vi "Main.vi"() -> ()   [LabVIEW 2019]
uses:
  Main_state_enum.ctl
  Uart_codes_enum.ctl
  <vilib>/Instr/_visa.llb/VISA Configure Serial Port (Instr).vi
  <vilib>/Utility/file.llb/Write Delimited Spreadsheet (string).vi
panel:
  out "Polling error tips":string
  out "Serial error tips":string
  out "Blocker":string
  out "File path":path
  in  "Seconds":i32 caption="s" min=0 max=59 step=1
  in  "Minutes":i32 caption="m" min=0 max=59 step=1
  in  "Hours":i32 caption="h" min=0 max=23 step=1
  out "Cycle string":string caption="Automatic polling interval"
  out "Next reading in":string
  in  "Demo":bool caption="Frige/Freezer critical failure demo"
  in  "Manual read":bool caption="Reset serial or filename"
  out "Slide":dbl(slide) scale=0.0..3.0
  out "Demo indicator":bool
  out "Freezer alarm":bool
  out "Fridge alarm":bool
  out "AVG":dbl format="%#_4g"
  in  "Continue":bool caption="Reset serial or filename"
  in  "Filename":string
  out "Trend graph":cluster{i32, dbl}[](graph) caption="Average indoors temperature (Last 30 readings)"
  out "Trend":dbl[](array[numeric])
  out "Fridge warning":string
  out "Freezer warning":string
  out "FreezerSTR":string caption="Freezer"
  out "FridgeSTR":string caption="Fridge"
  out "BathroomSTR":string caption="Bathroom"
  out "LivingroomSTR":string caption="Livingroom"
  out "BedroomSTR":string caption="Bedroom"
  out "KitchenSTR":string caption="Kitchen"
  out "Last reading":string
  out "Current time":string
  out "Freezer":dbl(slide) scale=-18.0..-10.0 scale format="%#_2g"
  out "Fridge":dbl(slide) scale=3.0..6.0
  out "Bathroom":dbl(slide) scale=16.0..30.0
  out "Livingroom":dbl(slide) scale=16.0..30.0
  out "Bedroom":dbl(slide) scale=16.0..30.0
  out "Kitchen":dbl(slide) scale=16.0..30.0
  out "Outdoors":dbl(slide) scale=-30.0..30.0
  out "Reading Cycle(s)":i32=15
  out "UI show array":dbl[](array[numeric])=[6.0, 13.0, 24.0, 20.0, 21.0, 24.0, 4.0, -17.0]
  in  "insert_comport":refnum<visa-resource-name>="COM5" caption="Serial port"
  out "csv save array":string[](array[string])
  in  "stop":bool
  out "OutdoorsSTR":string caption="Outdoors"
  out "Floorplan":picture
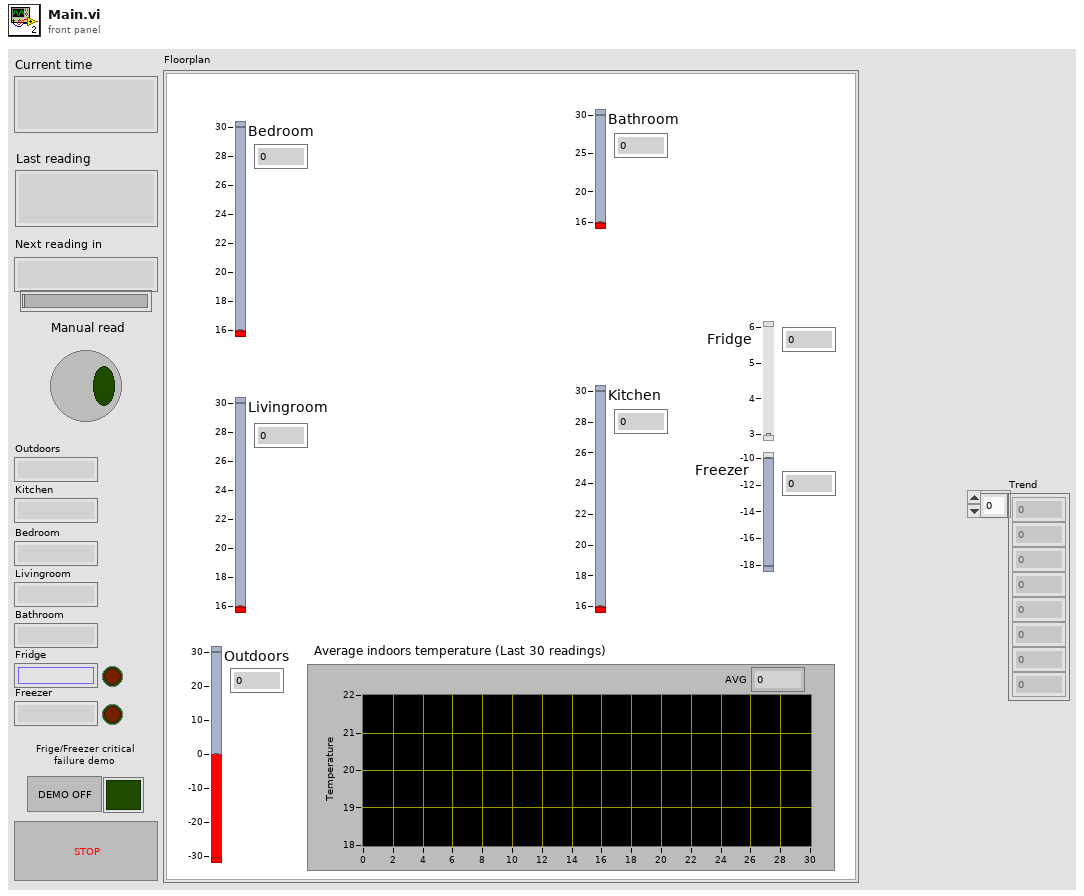
[diagram p1: front panel]
types:
  T1 = typedef "Uart_codes_enum.ctl" = enum16{"GET_READINGS", "FRIDGE_FREEZER_FAIL"}
  T2 = typedef "Main_state_enum.ctl" = enum16{"Init", "Set_startup_config", "Check_startup_config", "Read_serial", "Check_serial", "Update", "Wait"}
  T3 = enum8{"Enabled", "Disabled", "Disabled and Grayed Out"}
  T4 = typedef "imagedata.ctl" = cluster{"image type":i32, "image depth":i32, "image":u8[], "mask":u8[], "colors":u32[], "Rectangle":cluster{"left":i16, "top":i16, "right":i16, "bottom":i16}}
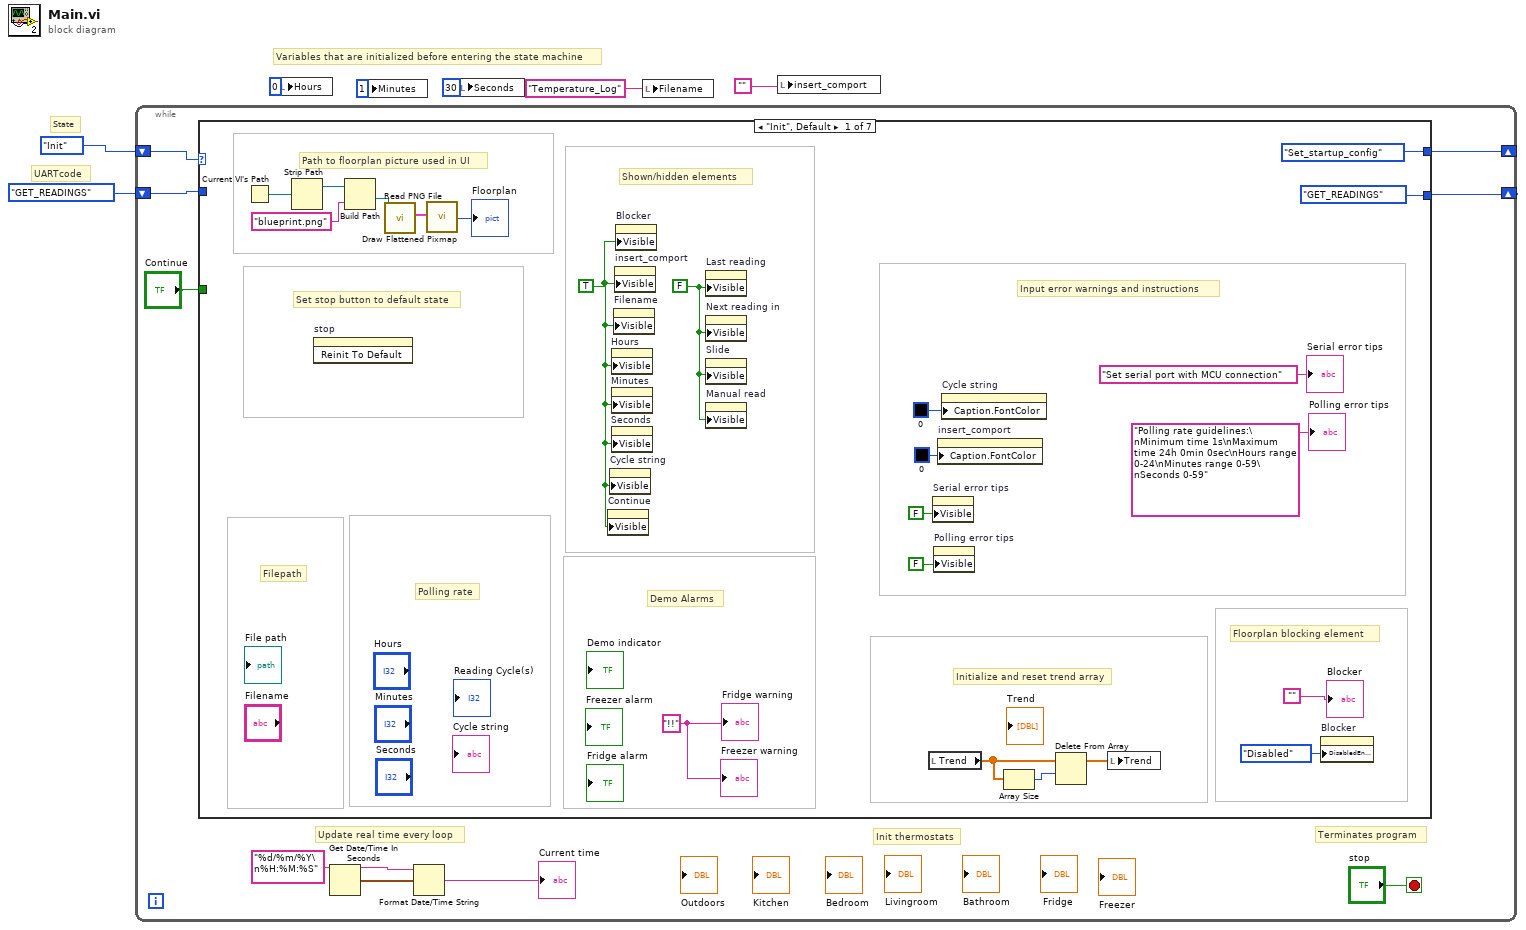
[diagram p0: block diagram]
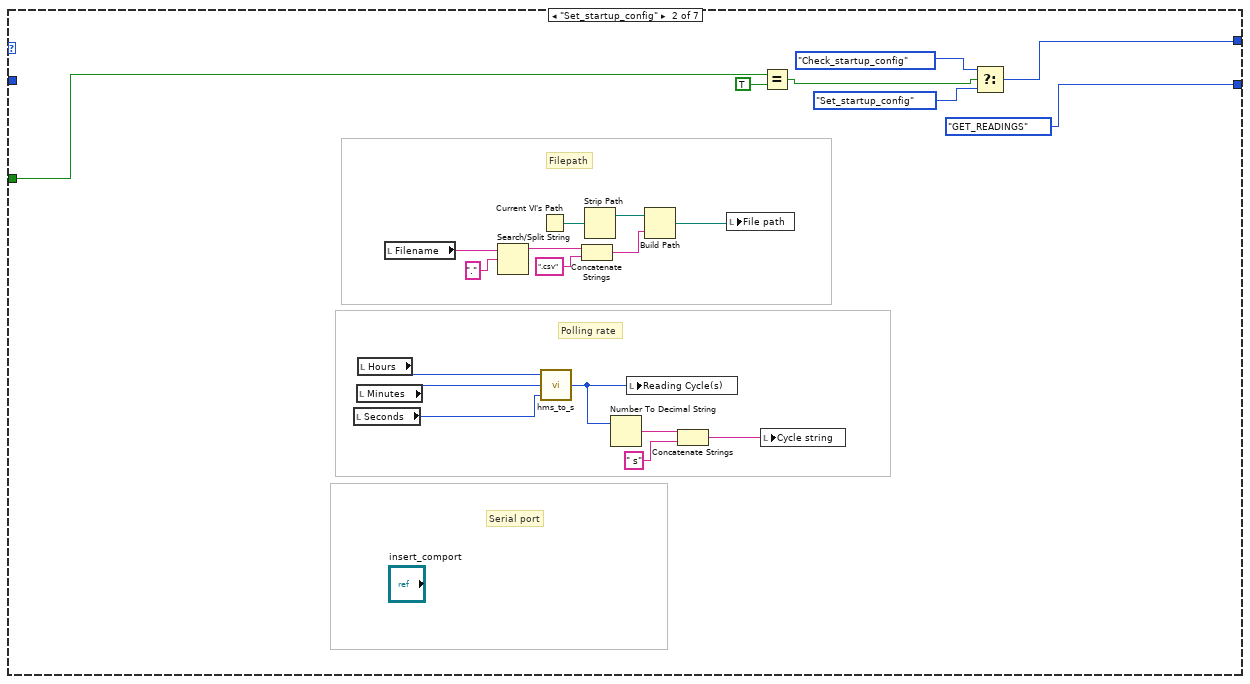
[diagram p2: hidden frame]
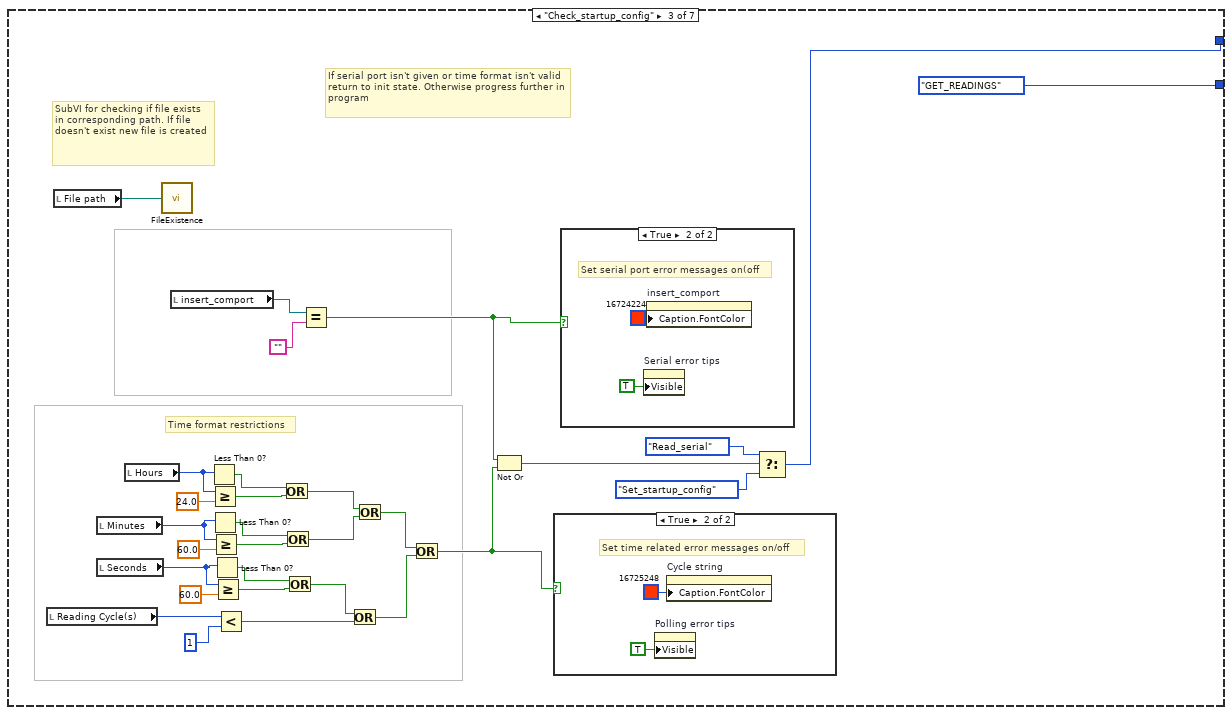
[diagram p3: hidden frame]
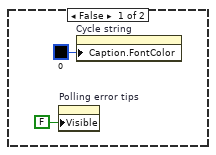
[diagram p4: hidden frame]
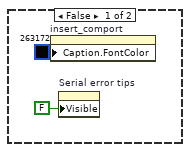
[diagram p5: hidden frame]
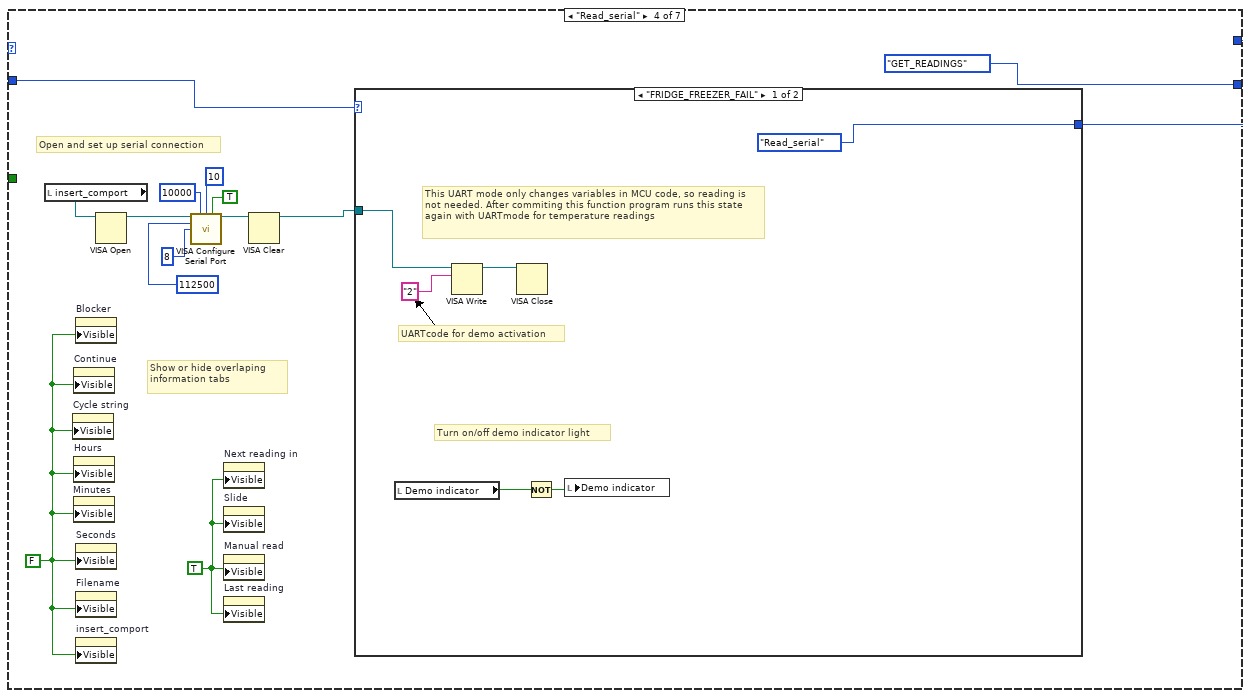
[diagram p6: hidden frame]
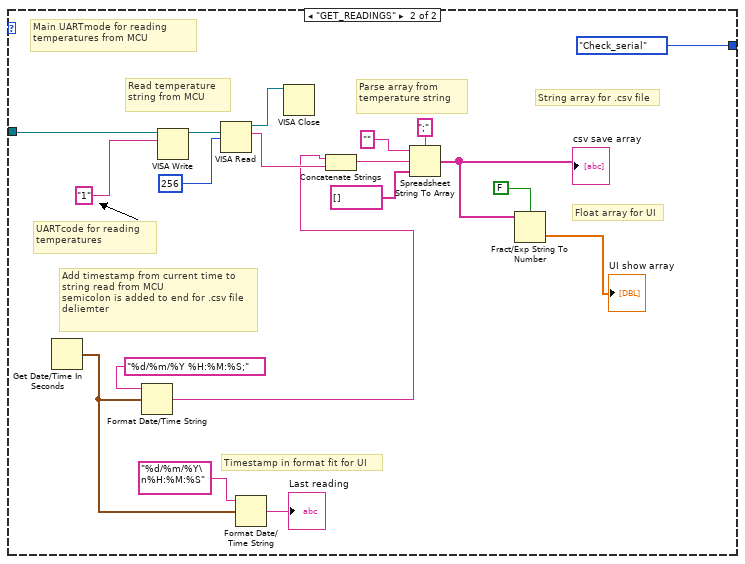
[diagram p7: hidden frame]
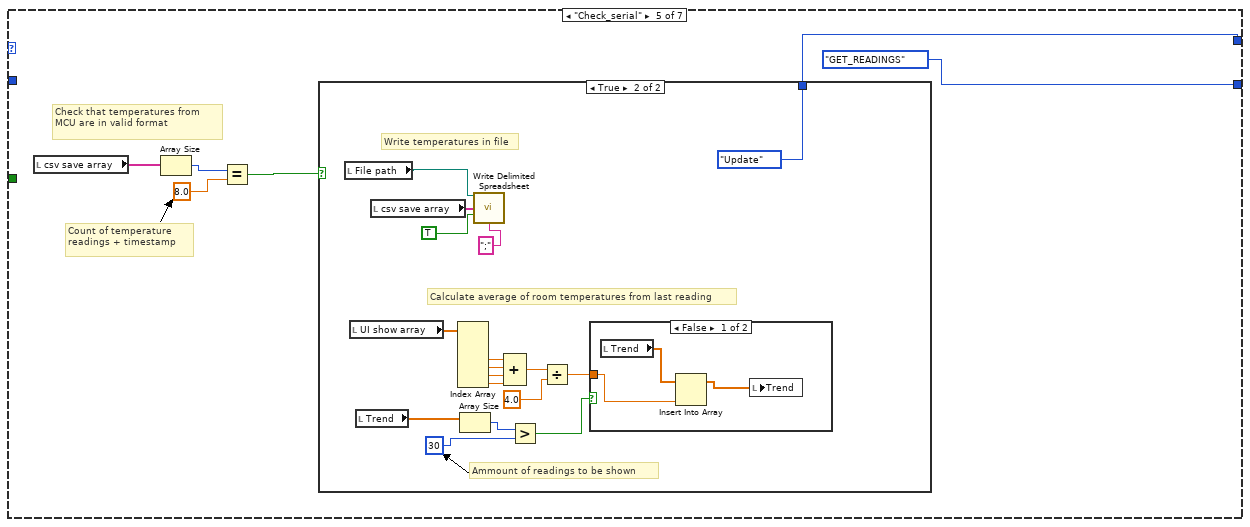
[diagram p8: hidden frame]
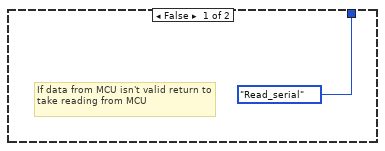
[diagram p9: hidden frame]
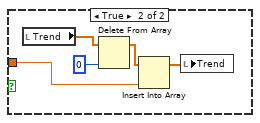
[diagram p10: hidden frame]
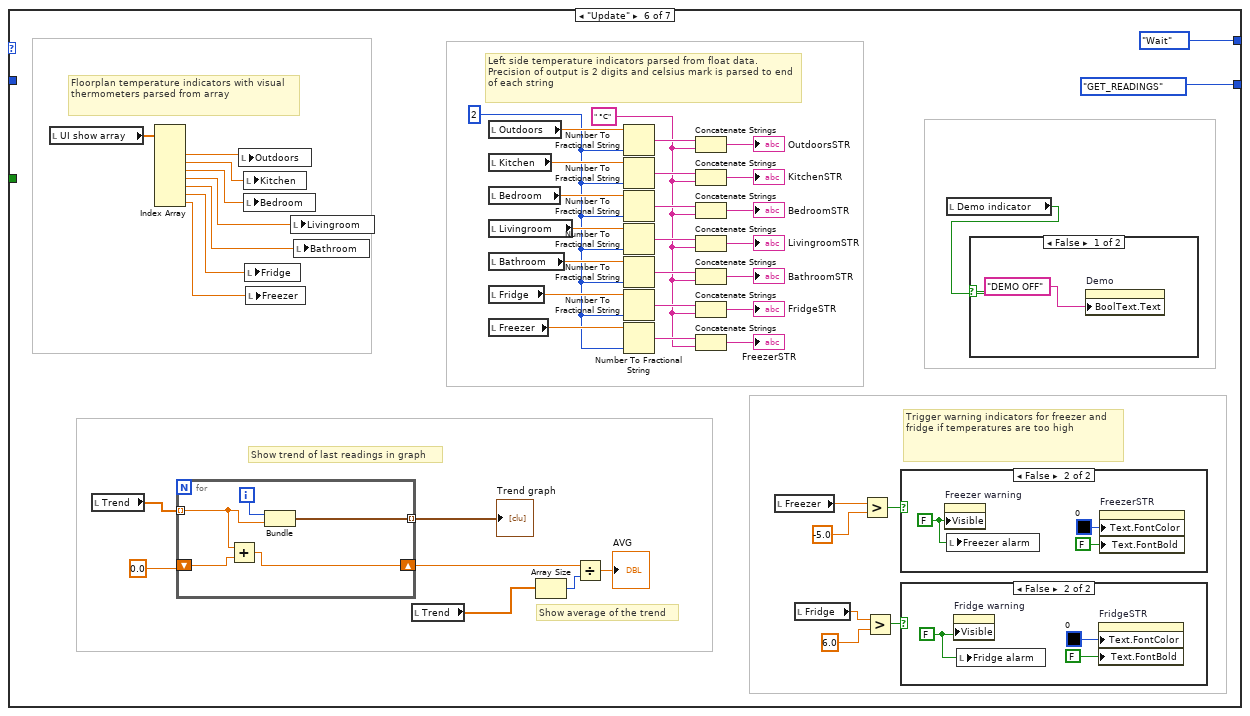
[diagram p11: hidden frame]
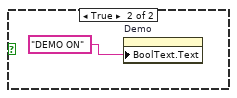
[diagram p12: hidden frame]
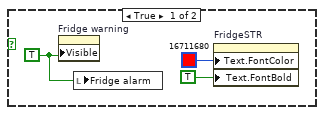
[diagram p13: hidden frame]
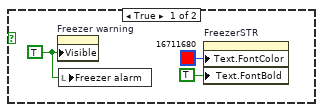
[diagram p14: hidden frame]
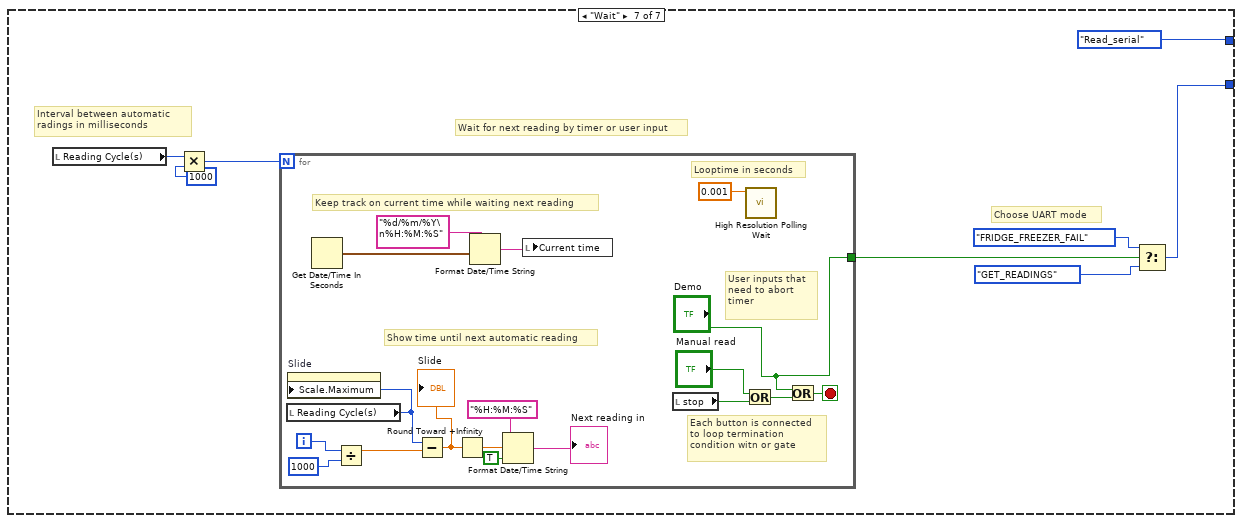
[diagram p15: hidden frame]
diagram:
  # "UARTcode"
  # "State"
  # "Variables that are initialized before entering the state machine"
  n1 = while {
    shift-right: [w15] -> _
    shift-left: Main_state_enum."Init" -> [w16]
    shift-right: [w11] -> _
    shift-left: Uart_codes_enum."GET_READINGS" -> [w12]
    stop <- "stop" stop-if-true
    # "Init thermostats"
    # "Terminates program"
    # "Update real time every loop"
    n2 = case shown="\"Init\", Default" w16 {
      tunnel: [Main_state_enum."Set_startup_config" w54 w88 w103 w140 Main_state_enum."Wait" Main_state_enum."Read_serial"] -> w15
      tunnel: w12 -> [_ _ _ w112 _ _ _]
      tunnel: [Uart_codes_enum."GET_READINGS" Uart_codes_enum."GET_READINGS" Uart_codes_enum."GET_READINGS" Uart_codes_enum."GET_READINGS" Uart_codes_enum."GET_READINGS" Uart_codes_enum."GET_READINGS" w240] -> w11
      tunnel: "Continue" -> [_ w60 _ _ _ _ _]
      frame "Init", Default {
        w17 = TRUE ("Visible")
        w27 = FALSE ("Visible")
        w34 = "!!" ("String 3")
        # "Floorplan blocking element"
        # "Input error warnings and instructions"
        # "Shown/hidden elements"
        # "Demo Alarms"
        # "Polling rate"
        # "Filepath"
        # "Set stop button to default state"
        # "Path to floorplan picture used in UI"
        # "Initialize and reset trend array"
        n3 = Current VI's Path() -> (path=w32:path)
        n4 = Strip Path(path=w32) -> (stripped path=w33:path)  [unwired: 1 out]
        n5 = invoke on="stop" class="Bool (strict)" method="Reinit To Default"() -> ()  [unwired: 3 in, 3 out]
        n6 = Build Path(base path=w33, name or relative path="blueprint.png") -> (appended path=w29:path)
        n7 = call <vilib>:"Read PNG File.vi"("path to PNG file"=w29) -> ("image data"=w30:T4)  [unwired: 8 in, 2 out]
        n8 = call <vilib>:"Draw Flattened Pixmap.vi"("image data"=w30) -> ("new picture"=→"Floorplan":picture)  [unwired: 8 in]
        n9 = property on="Continue" class="Bool"("Visible"=w17) -> ()  [unwired: 2 in, 2 out]
        n10 = property on="Cycle string" class="Str"("Visible"=w17) -> ()  [unwired: 2 in, 2 out]
        n11 = property on="Hours" class="DigNum (strict)"("Visible"=w17) -> ()  [unwired: 2 in, 2 out]
        n12 = property on="Minutes" class="DigNum (strict)"("Visible"=w17) -> ()  [unwired: 2 in, 2 out]
        n13 = property on="Seconds" class="DigNum (strict)"("Visible"=w17) -> ()  [unwired: 2 in, 2 out]
        n14 = property on="Filename" class="Str"("Visible"=w17) -> ()  [unwired: 2 in, 2 out]
        n15 = property on="insert_comport" class="VISAName"("Visible"=w17) -> ()  [unwired: 2 in, 2 out]
        n16 = property on="Blocker" class="Str"("Visible"=w17) -> ()  [unwired: 2 in, 2 out]
        n17 = property on="Last reading" class="Str"("Visible"=w27) -> ()  [unwired: 2 in, 2 out]
        n18 = property on="Next reading in" class="Str"("Visible"=w27) -> ()  [unwired: 2 in, 2 out]
        n19 = property on="Slide" class="Slide (strict)"("Visible"=w27) -> ()  [unwired: 2 in, 2 out]
        n20 = property on="Manual read" class="Bool"("Visible"=w27) -> ()  [unwired: 2 in, 2 out]
        n21 = local read "Trend"() -> (w37:dbl[])
        n22 = property on="Serial error tips" class="Str"("Visible"=FALSE) -> ()  [unwired: 2 in, 2 out]
        n23 = property on="Polling error tips" class="Str"("Visible"=FALSE) -> ()  [unwired: 2 in, 2 out]
        n24 = property on="insert_comport" class="VISAName"("Caption.FontColor"=u32 0 ("Caption.Font:Color")) -> ()  [unwired: 2 in, 2 out]
        n25 = property on="Cycle string" class="Str"("Caption.FontColor"=u32 0 ("Caption.Font:Color")) -> ()  [unwired: 2 in, 2 out]
        n26 = Array Size(array=w37) -> (size(s)=w35:i32)
        n27 = Delete From Array(array=w37, length=w35) -> (array with subset deleted=w36:dbl[])  [unwired: 1 in, 1 out]
        n28 = local write "Trend"(w36) -> ()
        n29 = property on="Blocker" class="Str"("DisabledEnum"=T3."Disabled" ("Disabled")) -> ()  [unwired: 2 in, 2 out]
        "Freezer warning" <- w34
        "Fridge warning" <- w34
        "Serial error tips" <- "Set serial port with MCU connection" ("Serial error tips")
        "Polling error tips" <- "Polling rate guidelines:\nMinimum time 1s\nMaximum time 24h 0min 0sec\nHours range 0-24\nMinutes range 0-59\nSeconds 0-59" ("Polling error tips")
        "Blocker" <- ""
      }
      frame "Set_startup_config" {
        # "Serial port"
        # "Polling rate"
        # "Filepath"
        n30 = local read "Seconds"() -> (w39:i32)
        n31 = local read "Minutes"() -> (w40:i32)
        n32 = local read "Hours"() -> (w41:i32)
        n33 = local read "Filename"() -> (w51:string)
        n34 = Search/Split String(string=w51, search string/char (-)=".") -> (substring before match=w50:string)  [unwired: 1 in, 2 out]
        n35 = Current VI's Path() -> (path=w48:path)
        n36 = call "hms_to_s.vi"("s"=w39, "m"=w40, "h"=w41) -> ("result"=w44:i32)
        n37 = Concatenate Strings(w50, ".csv" ("string")) -> (w49:string)
        n38 = Strip Path(path=w48) -> (stripped path=w47:path)  [unwired: 1 out]
        n39 = Number To Decimal String(number=w44) -> (decimal integer string=w53:string)  [unwired: 1 in]
        n40 = local write "Reading Cycle(s)"(w44) -> ()
        n41 = Build Path(base path=w47, name or relative path=w49) -> (appended path=w42:path)
        n42 = Concatenate Strings(w53, " s" ("string")) -> (w43:string)
        n43 = local write "File path"(w42) -> ()
        n44 = local write "Cycle string"(w43) -> ()
        n45 = Equal?(x=w60, y=TRUE) -> (x = y?=w58:bool)
        n46 = Select(t=Main_state_enum."Check_startup_config", s=w58, f=Main_state_enum."Set_startup_config") -> (s? t:f=w54:T2)
      }
      frame "Check_startup_config" {
        # "Time format restrictions"
        # "If serial port isn't given or time format isn't valid return to init state. Otherwise progress further in program"
        # "SubVI for checking if file exists in corresponding path. If file doesn't exist new file is created"
        n47 = local read "Reading Cycle(s)"() -> (w65:i32)
        n48 = local read "File path"() -> (w84:path)
        n49 = local read "Minutes"() -> (w73:i32)
        n50 = local read "Seconds"() -> (w72:i32)
        n51 = local read "Hours"() -> (w82:i32)
        n52 = call "FileExistence.vi"("Path"=w84) -> ()
        n53 = local read "insert_comport"() -> (w86:refnum<visa-resource-name>)
        n54 = Less Than 0?(x=w82) -> (x < 0?=w81:bool)
        n55 = Greater Or Equal?(x=w82, y=24.0) -> (x >= y?=w80:bool)
        n56 = Less Than 0?(x=w73) -> (x < 0?=w78:bool)
        n57 = Greater Or Equal?(x=w73, y=60.0) -> (x >= y?=w77:bool)
        n58 = Less Than 0?(x=w72) -> (x < 0?=w75:bool)
        n59 = Greater Or Equal?(x=w72, y=60.0) -> (x >= y?=w74:bool)
        n60 = Less?(x=w65, y=1) -> (x < y?=w63:bool)
        n61 = Or(x=w81, y=w80) -> (x .or. y?=w71:bool)
        n62 = Or(x=w78, y=w77) -> (x .or. y?=w70:bool)
        n63 = Or(x=w75, y=w74) -> (x .or. y?=w62:bool)
        n64 = Equal?(x=w86, y="") -> (x = y?=w67:bool)
        n65 = Or(x=w62, y=w63) -> (x .or. y?=w61:bool)
        n66 = Or(x=w71, y=w70) -> (x .or. y?=w69:bool)
        n67 = Or(x=w69, y=w61) -> (x .or. y?=w68:bool)
        n68 = Not Or(1:w68, 2:w67) -> (0:w66:bool)
        n69 = case shown="True" w68 {
          frame False {
            n70 = property on="Polling error tips" class="Str"("Visible"=FALSE) -> ()  [unwired: 2 in, 2 out]
            n71 = property on="Cycle string" class="Str"("Caption.FontColor"=u32 0 ("Caption.Font:Color")) -> ()  [unwired: 2 in, 2 out]
          }
          frame True {
            # "Set time related error messages on/off"
            n72 = property on="Polling error tips" class="Str"("Visible"=TRUE) -> ()  [unwired: 2 in, 2 out]
            n73 = property on="Cycle string" class="Str"("Caption.FontColor"=u32 16725248 ("Caption.Font:Color")) -> ()  [unwired: 2 in, 2 out]
          }
        }
        n74 = case shown="True" w67 {
          frame False {
            n75 = property on="insert_comport" class="VISAName"("Caption.FontColor"=u32 263172 ("Label.Font:Color")) -> ()  [unwired: 2 in, 2 out]
            n76 = property on="Serial error tips" class="Str"("Visible"=FALSE) -> ()  [unwired: 2 in, 2 out]
          }
          frame True {
            # "Set serial port error messages on(off"
            n77 = property on="Serial error tips" class="Str"("Visible"=TRUE) -> ()  [unwired: 2 in, 2 out]
            n78 = property on="insert_comport" class="VISAName"("Caption.FontColor"=u32 16724224 ("Label.Font:Color")) -> ()  [unwired: 2 in, 2 out]
          }
        }
        n79 = Select(t=Main_state_enum."Read_serial", s=w66, f=Main_state_enum."Set_startup_config") -> (s? t:f=w88:T2)
      }
      frame "Read_serial" {
        w101 = TRUE
        w99 = FALSE
        # "Open and set up serial connection"
        # "Show or hide overlaping information tabs"
        n80 = local read "insert_comport"() -> (w102:refnum<visa-resource-name>)
        n81 = property on="Cycle string" class="Str"("Visible"=w99) -> ()  [unwired: 2 in, 2 out]
        n82 = property on="Continue" class="Bool"("Visible"=w99) -> ()  [unwired: 2 in, 2 out]
        n83 = property on="Hours" class="DigNum (strict)"("Visible"=w99) -> ()  [unwired: 2 in, 2 out]
        n84 = property on="Minutes" class="DigNum (strict)"("Visible"=w99) -> ()  [unwired: 2 in, 2 out]
        n85 = property on="Blocker" class="Str"("Visible"=w99) -> ()  [unwired: 2 in, 2 out]
        n86 = property on="Seconds" class="DigNum (strict)"("Visible"=w99) -> ()  [unwired: 2 in, 2 out]
        n87 = property on="Filename" class="Str"("Visible"=w99) -> ()  [unwired: 2 in, 2 out]
        n88 = property on="insert_comport" class="VISAName"("Visible"=w99) -> ()  [unwired: 2 in, 2 out]
        n89 = VISA Open(VISA resource name=w102) -> (VISA resource name=w111:refnum<visa-resource-name>)  [unwired: 4 in, 1 out]
        n90 = call-poly "VISA Configure Serial Port"("VISA resource name"=w111, "timeout (10sec)"=u32 10000, "termination char\n(0xA = '\\n' = LF)"=u8 10 ("termination char\n(0xA = '\\n' = LF)"), "Enable Termination\nChar (T)"=TRUE ("Enable Termination\nChar (T)"), "baud rate (9600)"=u32 112500, "data bits (8)"=u16 8) -> ("VISA resource name out"=w110:refnum<visa-resource-name>)  [unwired: 8 in, 1 out]
        n91 = property on="Next reading in" class="Str"("Visible"=w101) -> ()  [unwired: 2 in, 2 out]
        n92 = property on="Slide" class="Slide (strict)"("Visible"=w101) -> ()  [unwired: 2 in, 2 out]
        n93 = property on="Manual read" class="Bool"("Visible"=w101) -> ()  [unwired: 2 in, 2 out]
        n94 = property on="Last reading" class="Str"("Visible"=w101) -> ()  [unwired: 2 in, 2 out]
        n95 = VISA Clear(VISA resource name=w110) -> (VISA resource name out=w104:refnum<visa-resource-name>)  [unwired: 1 in, 1 out]
        n96 = case shown="\"FRIDGE_FREEZER_FAIL\"" w112 {
          tunnel: w104 -> [w116 w126]
          tunnel: [Main_state_enum."Read_serial" Main_state_enum."Check_serial"] -> w103
          frame "FRIDGE_FREEZER_FAIL" {
            # "UARTcode for demo activation"
            # "This UART mode only changes variables in MCU code, so reading is not needed. After commiting this function program runs this state again with UARTmode for temperature readings"
            # "Turn on/off demo indicator light"
            n97 = local read "Demo indicator"() -> (w113:bool)
            n98 = VISA Write(VISA resource name=w116, write buffer="2") -> (VISA resource name out=w117:refnum<visa-resource-name>)  [unwired: 1 in, 2 out]
            n99 = VISA Close(VISA resource name=w117) -> ()  [unwired: 1 in, 1 out]
            n100 = Not(x=w113) -> (.not. x?=w114:bool)
            n101 = local write "Demo indicator"(w114) -> ()
          }
          frame "GET_READINGS" {
            # "Main UARTmode for reading temperatures from MCU"
            # "Parse array from temperature string"
            # "Float array for UI"
            # "String array for .csv file"
            # "Read temperature string from MCU"
            # "UARTcode for reading temperatures"
            # "Timestamp in format fit for UI"
            # "Add timestamp from current time to string read from MCU\nsemicolon is added to end for .csv file deliemter"
            n102 = Get Date/Time In Seconds() -> (seconds since 1Jan1904=w121:timestamp)
            n103 = Format Date/Time String(time format string (%c)="%d/%m/%Y %H:%M:%S;", seconds (now)=w121) -> (date/time string=w122:string)  [unwired: 1 in]
            n104 = VISA Write(VISA resource name=w126, write buffer="1") -> (VISA resource name out=w128:refnum<visa-resource-name>)  [unwired: 1 in, 2 out]
            n105 = VISA Read(VISA resource name=w128, byte count=u32 256) -> (VISA resource name out=w136:refnum<visa-resource-name>, read buffer=w131:string)  [unwired: 1 in, 2 out]
            n106 = Format Date/Time String(time format string (%c)="%d/%m/%Y\n%H:%M:%S", seconds (now)=w121) -> (date/time string=→"Last reading":string)  [unwired: 1 in]
            n107 = VISA Close(VISA resource name=w136) -> ()  [unwired: 1 in, 1 out]
            n108 = Concatenate Strings(w122, w131) -> (w130:string)
            n109 = Spreadsheet String To Array(delimiter (Tab)=";", format string="", spreadsheet string=w130, array type (2D Dbl)=string[] []) -> (array=w124:string[])
            "csv save array" <- w124
            n110 = Fract/Exp String To Number(use system decimal point (T)=FALSE, string=w124) -> (number=→"UI show array":dbl[])  [unwired: 2 in, 1 out]
          }
        }
      }
      frame "Check_serial" {
        # "Count of temperature readings + timestamp"
        # "Check that temperatures from MCU are in valid format"
        n111 = local read "csv save array"() -> (w139:string[])
        n112 = Array Size(array=w139) -> (size(s)=w142:i32)
        n113 = Equal?(x=w142, y=8.0) -> (x = y?=w141:bool)
        n114 = case shown="True" w141 {
          tunnel: [Main_state_enum."Read_serial" Main_state_enum."Update"] -> w140
          frame False {
            # "If data from MCU isn't valid return to take reading from MCU"
          }
          frame True {
            # "Write temperatures in file"
            # "Ammount of readings to be shown"
            # "Calculate average of room temperatures from last reading"
            n115 = local read "File path"() -> (w145:path)
            n116 = local read "UI show array"() -> (w156:dbl[])
            n117 = local read "Trend"() -> (w158:dbl[])
            n118 = local read "csv save array"() -> (w161:string[])
            n119 = Index Array(array=w156) -> (element #3=w155:dbl, element #4=w154:dbl, element #5=w153:dbl, element #6=w152:dbl)  [unwired: 6 in, 2 out]
            n120 = Array Size(array=w158) -> (size(s)=w157:i32)
            n121 = call-poly <vilib>:"Write Delimited Spreadsheet.vi"("file path (dialog if empty)"=w145, "1D data"=w161, "append to file? (new file:F)"=TRUE, "delimiter (\\t)"=";" ("delimiter (\\t)")) -> ()  [unwired: 10 in, 2 out]
            n122 = Compound Arithmetic op=ADD(w155, w154, w153, w152) -> (w151:dbl)
            n123 = Greater?(x=w157, y=30) -> (0:w150:bool)
            n124 = Divide(x=w151, y=4.0) -> (x/y=w149:dbl)
            n125 = case shown="False" w150 {
              tunnel: w149 -> [w164 w169]
              frame False {
                n126 = local read "Trend"() -> (w163:dbl[])
                n127 = Insert Into Array(array=w163, new element=w164) -> (w162:dbl[])  [unwired: 1 in]
                n128 = local write "Trend"(w162) -> ()
              }
              frame True {
                n129 = local read "Trend"() -> (w168:dbl[])
                n130 = Delete From Array(array=w168, index=0) -> (array with subset deleted=w166:dbl[])  [unwired: 1 in, 1 out]
                n131 = Insert Into Array(array=w166, new element=w169) -> (w165:dbl[])  [unwired: 1 in]
                n132 = local write "Trend"(w165) -> ()
              }
            }
          }
        }
      }
      frame "Update" {
        w187 = i16 2 ("precision (6)")
        w186 = " °C" ("string")
        # "Show average of the trend"
        # "Show trend of last readings in graph"
        # "Trigger warning indicators for freezer and fridge if temperatures are too high"
        # "Floorplan temperature indicators with visual thermometers parsed from array"
        # "Left side temperature indicators parsed from float data. Precision of output is 2 digits and celsius mark is parsed to end of each string"
        n133 = local read "UI show array"() -> (w216:dbl[])
        n134 = local read "Trend"() -> (w179:dbl[])
        n135 = Index Array(array=w216) -> (element #2=w215:dbl, element #3=w214:dbl, element #4=w213:dbl, element #5=w212:dbl, element #6=w211:dbl, element #7=w210:dbl, element #8=w209:dbl)  [unwired: 8 in, 1 out]
        n136 = for {
          tunnel: w179 -> [w221] mode=indexing
          tunnel: [w223] -> w178 mode=indexing
          shift-right: [w219] -> w176
          shift-left: 0.0 -> [w222]
          i -> [w220]
          n137 = Add(x=w221, y=w222) -> (x+y=w219:dbl)
          n138 = Bundle(w220, w221) -> (w223:cluster{i32, dbl})  [unwired: 1 in]
        }
        "Trend graph" <- w178
        n139 = local write "Outdoors"(w215) -> ()
        n140 = local write "Kitchen"(w214) -> ()
        n141 = local write "Bedroom"(w213) -> ()
        n142 = local write "Fridge"(w210) -> ()
        n143 = local write "Freezer"(w209) -> ()
        n144 = local write "Livingroom"(w212) -> ()
        n145 = local write "Bathroom"(w211) -> ()
        n146 = local read "Trend"() -> (w173:dbl[])
        n147 = local read "Outdoors"() -> (w208:dbl)
        n148 = local read "Kitchen"() -> (w193:dbl)
        n149 = local read "Bedroom"() -> (w192:dbl)
        n150 = local read "Livingroom"() -> (w191:dbl)
        n151 = local read "Bathroom"() -> (w190:dbl)
        n152 = local read "Fridge"() -> (w189:dbl)
        n153 = local read "Freezer"() -> (w188:dbl)
        n154 = Array Size(array=w173) -> (size(s)=w174:i32)
        n155 = Divide(x=w176, y=w174) -> (x/y=→"AVG":dbl)
        n156 = Number To Fractional String(number=w208, precision (6)=w187) -> (F-format string=w207:string)  [unwired: 2 in]
        n157 = Number To Fractional String(number=w193, precision (6)=w187) -> (F-format string=w205:string)  [unwired: 2 in]
        n158 = Number To Fractional String(number=w192, precision (6)=w187) -> (F-format string=w203:string)  [unwired: 2 in]
        n159 = Number To Fractional String(number=w191, precision (6)=w187) -> (F-format string=w201:string)  [unwired: 2 in]
        n160 = Number To Fractional String(number=w190, precision (6)=w187) -> (F-format string=w199:string)  [unwired: 2 in]
        n161 = Number To Fractional String(number=w189, precision (6)=w187) -> (F-format string=w197:string)  [unwired: 2 in]
        n162 = Number To Fractional String(number=w188, precision (6)=w187) -> (F-format string=w195:string)  [unwired: 2 in]
        n163 = Concatenate Strings(w207, w186) -> (→"OutdoorsSTR":string)
        n164 = Concatenate Strings(w205, w186) -> (→"KitchenSTR":string)
        n165 = Concatenate Strings(w203, w186) -> (→"BedroomSTR":string)
        n166 = Concatenate Strings(w201, w186) -> (→"LivingroomSTR":string)
        n167 = Concatenate Strings(w199, w186) -> (→"BathroomSTR":string)
        n168 = Concatenate Strings(w197, w186) -> (→"FridgeSTR":string)
        n169 = Concatenate Strings(w195, w186) -> (→"FreezerSTR":string)
        n170 = local read "Freezer"() -> (w184:dbl)
        n171 = local read "Fridge"() -> (w181:dbl)
        n172 = Greater?(x=w184, y=-5.0) -> (0:w183:bool)
        n173 = Greater?(x=w181, y=6.0) -> (0:w182:bool)
        n174 = case shown="False" w183 {
          frame True {
            w230 = TRUE ("Visible")
            n175 = property on="Freezer warning" class="Str"("Visible"=w230) -> ()  [unwired: 2 in, 2 out]
            n176 = local write "Freezer alarm"(w230) -> ()
            n177 = property on="FreezerSTR" class="Str"("Text.FontColor"=u32 16711680 ("Text.Font:Color"), "Text.FontBold"=TRUE ("Text.Font:Bold")) -> ()  [unwired: 2 in, 2 out]
          }
          frame False {
            w233 = FALSE ("Visible")
            n178 = property on="Freezer warning" class="Str"("Visible"=w233) -> ()  [unwired: 2 in, 2 out]
            n179 = local write "Freezer alarm"(w233) -> ()
            n180 = property on="FreezerSTR" class="Str"("Text.FontColor"=u32 0 ("Text.Font:Color"), "Text.FontBold"=FALSE ("Text.Font:Bold")) -> ()  [unwired: 2 in, 2 out]
          }
        }
        n181 = case shown="False" w182 {
          frame True {
            w224 = TRUE ("Visible")
            n182 = property on="Fridge warning" class="Str"("Visible"=w224) -> ()  [unwired: 2 in, 2 out]
            n183 = local write "Fridge alarm"(w224) -> ()
            n184 = property on="FridgeSTR" class="Str"("Text.FontColor"=u32 16711680 ("Text.Font:Color"), "Text.FontBold"=TRUE ("Text.Font:Bold")) -> ()  [unwired: 2 in, 2 out]
          }
          frame False {
            w227 = FALSE ("Visible")
            n185 = property on="Fridge warning" class="Str"("Visible"=w227) -> ()  [unwired: 2 in, 2 out]
            n186 = local write "Fridge alarm"(w227) -> ()
            n187 = property on="FridgeSTR" class="Str"("Text.FontColor"=u32 0 ("Text.Font:Color"), "Text.FontBold"=FALSE ("Text.Font:Bold")) -> ()  [unwired: 2 in, 2 out]
          }
        }
        n188 = local read "Demo indicator"() -> (w172:bool)
        n189 = case shown="False" w172 {
          frame False {
            n190 = property on="Demo" class="Bool"("BoolText.Text"="DEMO OFF" ("Boolean Text.Text")) -> ()  [unwired: 2 in, 2 out]
          }
          frame True {
            n191 = property on="Demo" class="Bool"("BoolText.Text"="DEMO ON" ("Boolean Text.Text")) -> ()  [unwired: 2 in, 2 out]
          }
        }
      }
      frame "Wait" {
        # "Choose UART mode"
        # "Interval between automatic radings in milliseconds"
        # "Wait for next reading by timer or user input"
        n192 = local read "Reading Cycle(s)"() -> (w243:i32)
        n193 = Multiply(x=w243, y=1000) -> (x*y=w242:i32)
        n194 = for {
          N: w242 -> [_]
          tunnel: ["Demo"] -> w237
          i -> [w256]
          stop <- w253 stop-if-true
          # "Each button is connected to loop termination condition witn or gate"
          # "User inputs that need to abort timer"
          # "Looptime in seconds"
          # "Keep track on current time while waiting next reading"
          # "Show time until next automatic reading"
          n195 = local read "Reading Cycle(s)"() -> (w244:i32)
          n196 = property on="Slide" class="Slide (strict)"("Scale.Maximum"=w244) -> ()  [unwired: 2 in, 2 out]
          n197 = Get Date/Time In Seconds() -> (seconds since 1Jan1904=w260:timestamp)
          n198 = Divide(x=w256, y=1000) -> (x/y=w255:dbl)
          n199 = Subtract(x=w244, y=w255) -> (x-y=w246:dbl)
          "Slide" <- w246
          n200 = Round Toward +Infinity(x=w246) -> (ceil(x): smallest int >= x=w250:dbl)
          n201 = Format Date/Time String(time format string (%c)="%d/%m/%Y\n%H:%M:%S", seconds (now)=w260) -> (date/time string=w258:string)  [unwired: 1 in]
          n202 = Format Date/Time String(time format string (%c)="%H:%M:%S", seconds (now)=w250, UTC format=TRUE) -> (date/time string=→"Next reading in":string)
          n203 = local write "Current time"(w258) -> ()
          n204 = local read "stop"() -> (w251:bool)
          n205 = Or(x="Manual read", y=w251) -> (x .or. y?=w252:bool)
          n206 = call <vilib>:"High Resolution Polling Wait.vi"("seconds to wait"=0.001) -> ()  [unwired: 10 in, 1 out]
          n207 = Or(x="Demo", y=w252) -> (x .or. y?=w253:bool)
        }
        n208 = Select(t=Uart_codes_enum."FRIDGE_FREEZER_FAIL", s=w237, f=Uart_codes_enum."GET_READINGS") -> (s? t:f=w240:T1)
      }
    }
    n209 = Get Date/Time In Seconds() -> (seconds since 1Jan1904=w14:timestamp)
    n210 = Format Date/Time String(time format string (%c)="%d/%m/%Y\n%H:%M:%S", seconds (now)=w14) -> (date/time string=→"Current time":string)  [unwired: 1 in]
  }
  n211 = local write "Hours"(0 ("h")) -> ()
  n212 = local write "Minutes"(1 ("m")) -> ()
  n213 = local write "Seconds"(30 ("s")) -> ()
  n214 = local write "Filename"("Temperature_Log" ("Filename")) -> ()
  n215 = local write "insert_comport"("") -> ()
